vi "Main.vi"(11 "Module Admin":refnum<class "Delacor_lib_QMH_Module Admin.lvclass">) -> ()   [LabVIEW 2025, in "Automatic Teller Machine (ATM).lvlib"]
doc: "This template is based off of the Queued Message Handler design pattern and the Queued Message Handler project template that ships with LabVIEW.\n\nThe main difference is that the queue is private to this module and communication between modules is performed via Broadcast and Request events.\n\nRequest events are wrapped in public API methods and are handled in the Event Handling Loop (EHL) of this VI. Any module can register for Broadcast events sent by this module. The EHL generates messages based on user interface actions.\n\nThe Message Handling Loop (MHL) processes messages generated by the EHL, or by other messages. The messages are string values, so new messages can be added easily to the Message Cases case structure in the MHL. Each message cluster can also provide an optional value for Message Data, which is a variant that can be converted to whatever message-specific data is required.\n_____\nBased on DQMH Dev Tools: Project Template 7.1.0.1503."
uses:
  Automatic Teller Machine (ATM).lvlib
  <vilib>/Delacor/Delacor QMH/Libraries/Module Admin_class/Delacor_lib_QMH_Module Admin.lvclass
  Module Data--cluster.ctl
  <vilib>/Delacor/Delacor QMH/Libraries/Message Queue_class/Delacor_lib_QMH_Message Queue.lvclass/Delacor_lib_QMH_Message Queue.ctl
  Stop Argument--cluster.ctl
  <vilib>/Delacor/Delacor QMH/Libraries/Module Admin_class/Delacor_lib_QMH_Module Admin.lvclass/Delacor_lib_QMH_Module Admin.ctl
  Reset Timer Argument--cluster.ctl
  <vilib>/Utility/miscctls.llb/LVPointTypeDef.ctl
  <vilib>/Delacor/Delacor QMH/Libraries/Message Queue_class/Delacor_lib_QMH_Enqueue Message (Single).vi
  <vilib>/Delacor/Delacor QMH/Libraries/Module Admin_class/Delacor_lib_QMH_Get External Launch.vi
  <vilib>/Delacor/Delacor QMH/Libraries/Message Queue_class/Delacor_lib_QMH_Message Queue.lvclass
panel:
  in  "Enter":bool
  in  "User Input":string
  in  "Right Buttons":T1
  out "Right Menu":T2
  in  "Left Buttons":T1
  out "Left Menu":T2
  in  "Card Simulator":bool
  out "ATM Messages":string
  out "error out":errorcluster
  out "Status":string
  in  "Simulate MHL Error":bool
  in  "Simulate EHL Error":bool
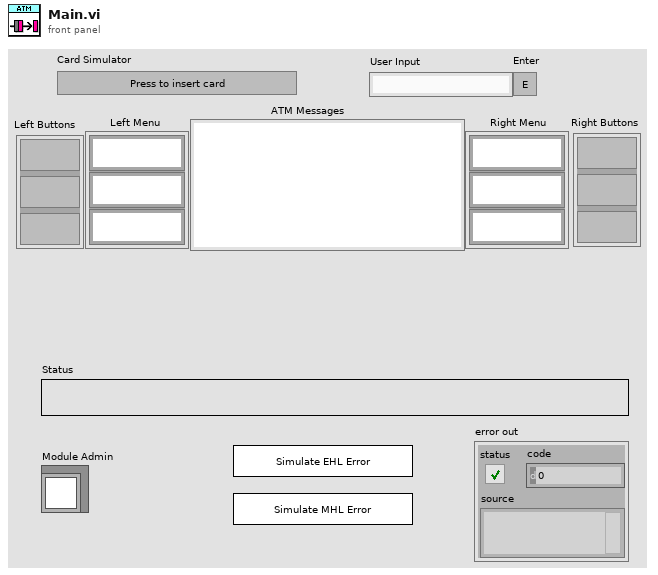
[diagram p1: front panel]
types:
  T1 = cluster{"Func Button":bool, "Func Button 2":bool, "Func Button 3":bool}
  T2 = cluster{"RFS String":string, "RFS String 2":string, "RFS String 3":string}
  T3 = typedef "Automatic Teller Machine (ATM).lvlib/Request Events--cluster.ctl" = cluster{"Stop Module":refnum<user-event>, "Show Panel":refnum<user-event>, "Hide Panel":refnum<user-event>, "Get Module Execution Status":refnum<user-event>, "Show Diagram":refnum<user-event>, "Private.Reset Timer":refnum<user-event>}
  T4 = typedef "Automatic Teller Machine (ATM).lvlib/Module Data--cluster.ctl" = cluster{"Status":string}
  T5 = enum32{"invalid lock state", "Not Locked", "Locked (No Password)", "Password-protected"}
  T6 = typedef "Automatic Teller Machine (ATM).lvlib/Stop Argument--cluster.ctl" = cluster{"Origin":string, "Exit via Stop Module Req?":bool, "Wait for Module to stop?":bool}
  T7 = typedef "Automatic Teller Machine (ATM).lvlib/Reset Timer Argument--cluster.ctl" = cluster{"Boolean":bool}
  T8 = typedef "LVPointTypeDef.ctl" = cluster{"Horizontal":i16, "Vertical":i16}
  T9 = enum32{"Invalid", "Standard", "Closed", "Hidden", "Minimized", "Maximized"}
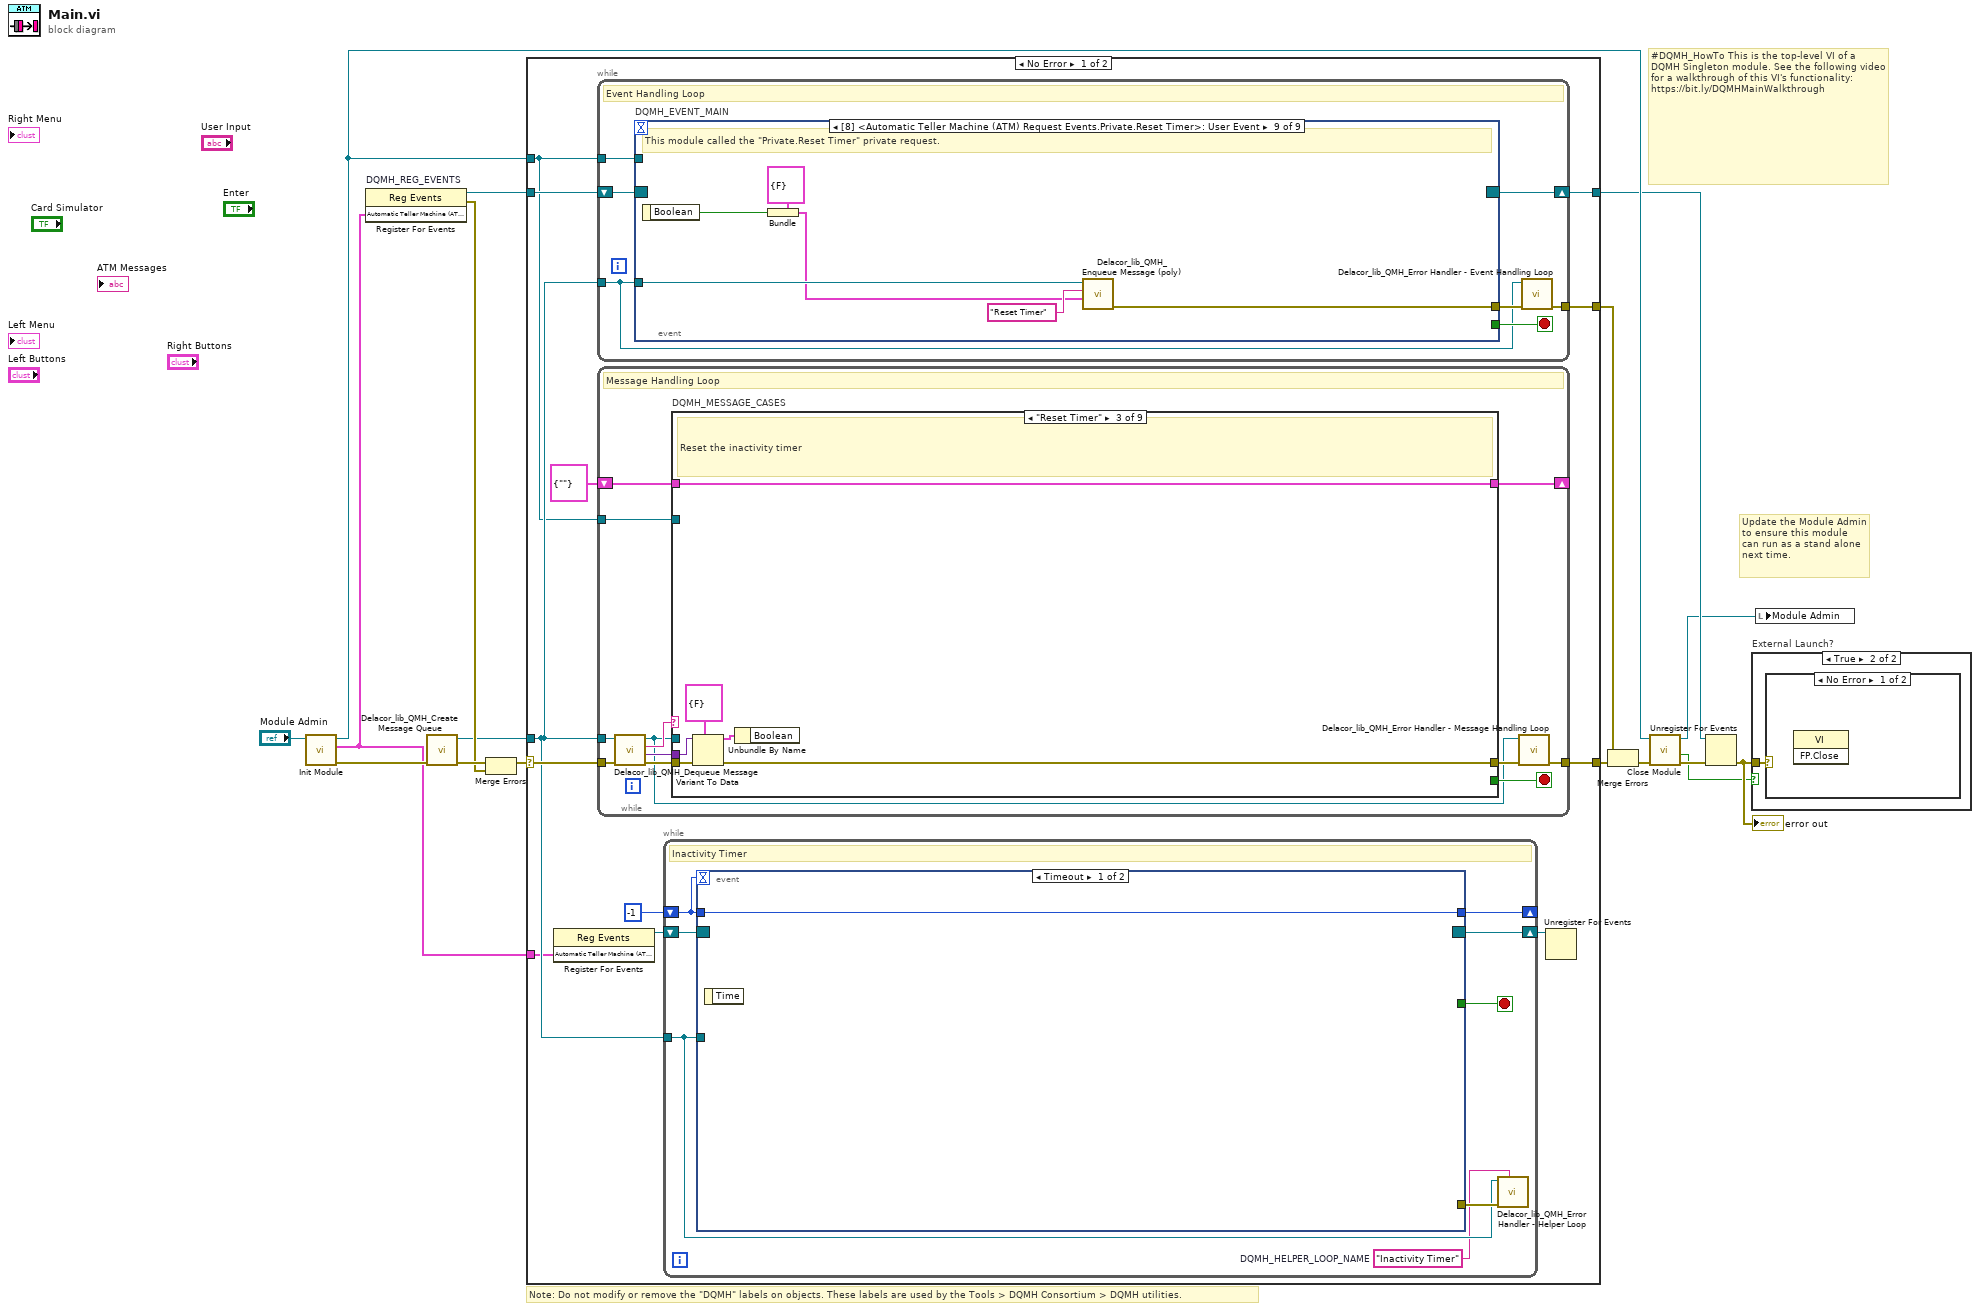
[diagram p0: block diagram]
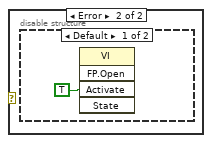
[diagram p3: hidden frame]
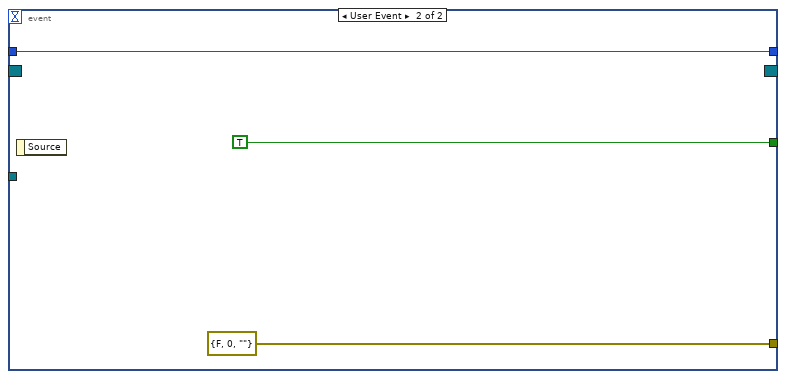
[diagram p5: hidden frame]
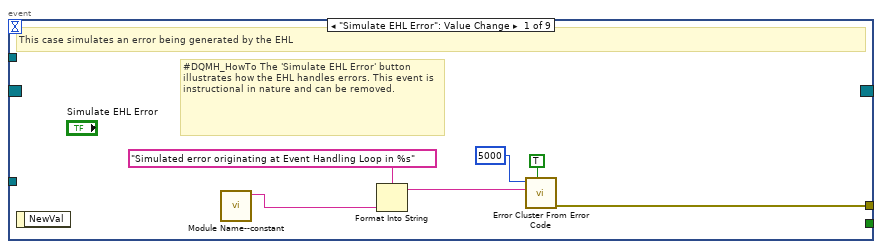
[diagram p6: hidden frame]
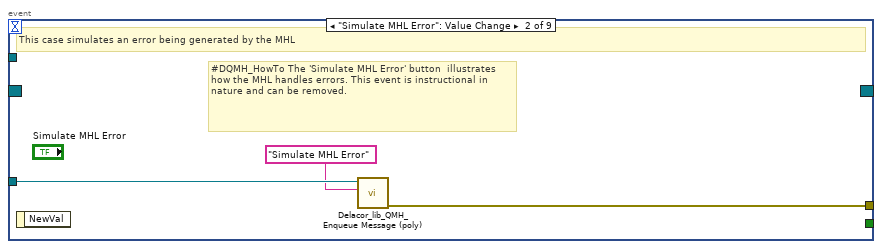
[diagram p7: hidden frame]
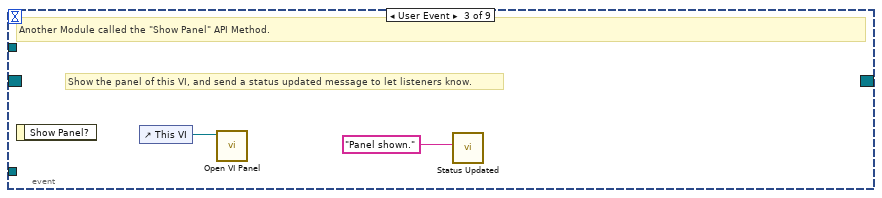
[diagram p8: hidden frame]
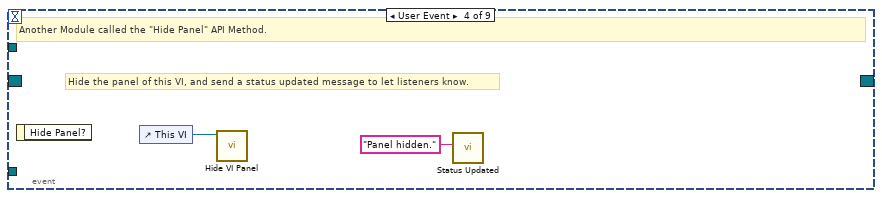
[diagram p9: hidden frame]
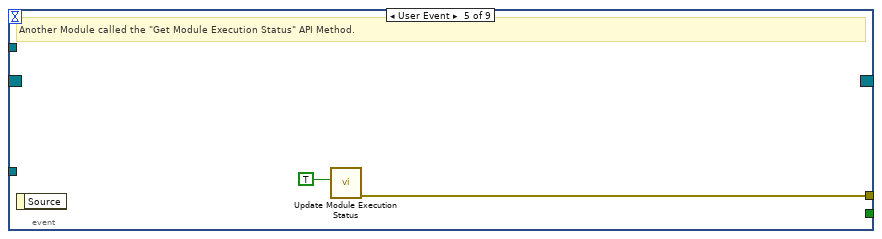
[diagram p10: hidden frame]
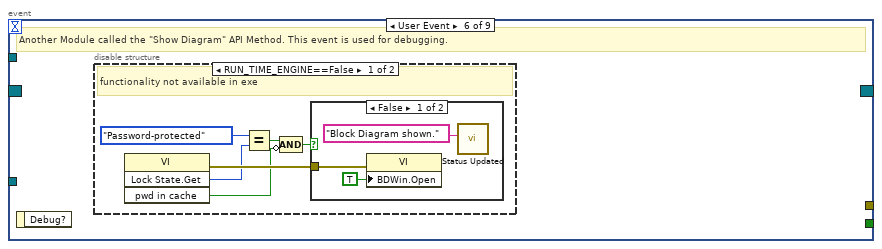
[diagram p11: hidden frame]
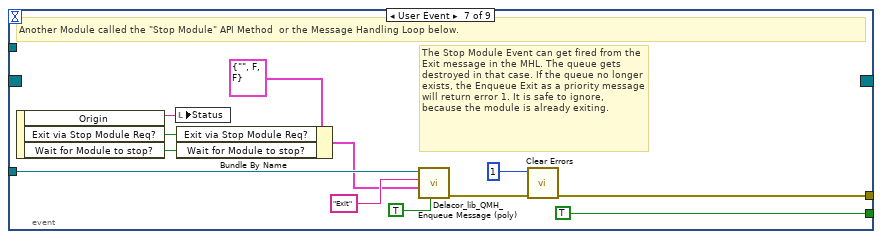
[diagram p14: hidden frame]
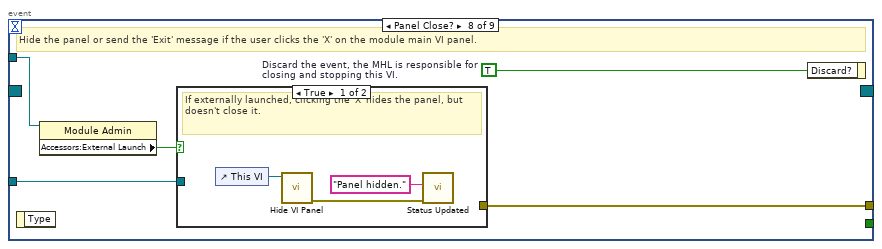
[diagram p15: hidden frame]
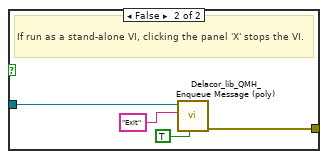
[diagram p16: hidden frame]
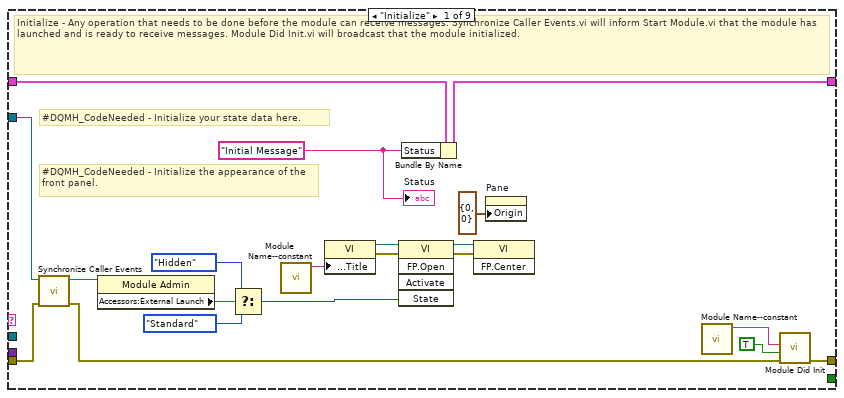
[diagram p17: hidden frame]
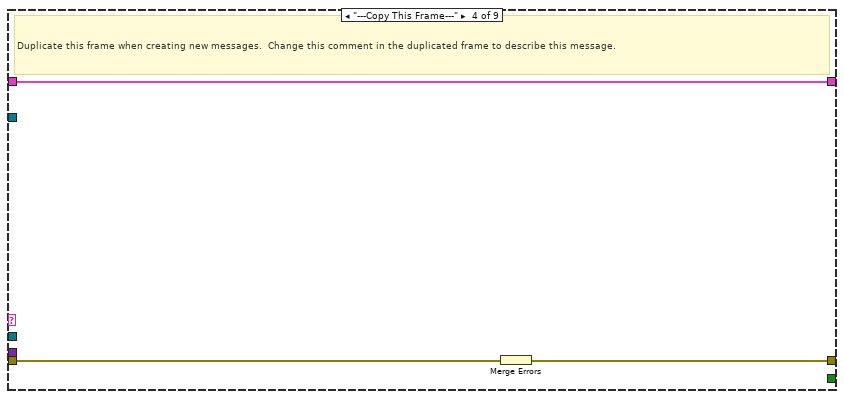
[diagram p19: hidden frame]
diagram:
  # "#DQMH_HowTo This is the top-level VI of a DQMH Singleton module. See the following video for a walkthrough of this VI's functionality: https://bit.ly/DQMHMainWalkthrough"
  # "Note: Do not modify or remove the \"DQMH\" labels on objects. These labels are used by the Tools > DQMH Consortium > DQMH utilities."
  # "Update the Module Admin to ensure this module can run as a stand alone next time."
  n1 = call "Init Module.vi"("Singleton Module Admin in"="Module Admin") -> ("error out"=w16:errorcluster, "Automatic Teller Machine (ATM) Request Events"=w1:T3, "Singleton Module Admin out"=w8:refnum<class "Delacor_lib_QMH_Module Admin.lvclass">)  [unwired: 8 in]
  n2 = register-events "DQMH_REG_EVENTS"(w1) -> (reference out=w6:refnum<event-registration>, error out=w9:errorcluster)  [unwired: 2 in]
  n3 = call <vilib>:"Delacor_lib_QMH_Create Message Queue.vi"("error in"=w16) -> ("error out"=w11:errorcluster, "Message Queue"=w5:refnum<class "Delacor_lib_QMH_Message Queue.lvclass">)  [unwired: 9 in]
  n4 = Merge Errors(w11, w9) -> (w10:errorcluster)
  n5 = case shown="No Error" w10 {
    selector: w10 -> [w27 w206]
    tunnel: [w29 w205] -> w17
    tunnel: [w26 w204] -> w7
    tunnel: w6 -> [w24 w204]
    tunnel: w5 -> [w23 w199]
    tunnel: [w28 _] -> w14
    tunnel: w8 -> [w22 w200]
    tunnel: w1 -> [w21 _]
    frame No Error {
      n6 = register-events ("DQMH_HELPER_REGFOREVENTS")(w21) -> (reference out=w19:refnum<event-registration>)  [unwired: 2 in, 1 out]
      n7 = while {
        tunnel: w23 -> [w42]
        shift-right: [w45] -> w26
        shift-left: w24 -> [w46]
        tunnel: [w47] -> w28
        tunnel: w22 -> [w43]
        stop <- w44 stop-if-true
        # "Event Handling Loop"
        n8 = event "DQMH_EVENT_MAIN" shown="[8] <Automatic Teller Machine (ATM) Request Events.Private.Reset Timer>: User Event" {
          selector: w46 -> [_ _ _ _ _ _ _ _ _]
          dyn-events: [_ _ _ _ _ _ _ _ _] -> w45
          timeout: _ -> [_ _ _ _ _ _ _ _ _]
          tunnel: [_ _ _ _ _ _ TRUE ("Discard?") _ _] -> w44
          tunnel: w42 -> [_ w56 _ _ _ _ w80 w87 w102]
          tunnel: [w54 w57 _ _ w63 _ w83 w89 w97] -> w48
          tunnel: w43 -> [_ _ _ _ _ _ _ w86 _]
          event "Simulate EHL Error": Value Change {
            # "#DQMH_HowTo The 'Simulate EHL Error' button  illustrates how the EHL handles errors. This event is instructional in nature and can be removed."
            # "This case simulates an error being generated by the EHL"
            n9 = event-data() -> ()  [unwired: 1 in, 1 out]
            n10 = call "Module Name--constant.vi"() -> ("Module Name"=w51:string)  [unwired: 11 in]
            n11 = Format Into String(format string="Simulated error originating at Event Handling Loop in %s", w51) -> (resulting string=w52:string)  [unwired: 2 in, 1 out]
            n12 = call <vilib>:"Error Cluster From Error Code.vi"("show call chain? (False)"=TRUE, "error message (\"\")"=w52, "error code (0)"=5000) -> ("error out"=w54:errorcluster)  [unwired: 6 in]
          }
          event "Simulate MHL Error": Value Change {
            # "#DQMH_HowTo The 'Simulate MHL Error' button  illustrates how the MHL handles errors. This event is instructional in nature and can be removed."
            # "This case simulates an error being generated by the MHL"
            n13 = event-data() -> ()  [unwired: 1 in, 1 out]
            n14 = call-poly <vilib>:"Delacor_lib_QMH_Enqueue Message (poly).vi"("Message"="Simulate MHL Error", "Message Queue in"=w56) -> ("error out"=w57:errorcluster)  [unwired: 8 in, 1 out]
          }
          event User Event {
            # "Show the panel of this VI, and send a status updated message to let listeners know."
            # "Another Module called the \"Show Panel\" API Method."
            n15 = event-data() -> ()  [unwired: 1 in, 1 out]
            n16 = control-ref of="This VI"() -> (w59:refnum<vi>)
            n17 = call "Open VI Panel.vi"("VI"=w59) -> ()  [unwired: 10 in, 1 out]
            n18 = call "Status Updated.vi"("Status"="Panel shown." ("format string")) -> ()  [unwired: 10 in, 1 out]
          }
          event User Event {
            # "Hide the panel of this VI, and send a status updated message to let listeners know."
            # "Another Module called the \"Hide Panel\" API Method."
            n19 = event-data() -> ()  [unwired: 1 in, 1 out]
            n20 = control-ref of="This VI"() -> (w61:refnum<vi>)
            n21 = call "Hide VI Panel.vi"("VI"=w61) -> ()  [unwired: 10 in, 1 out]
            n22 = call "Status Updated.vi"("Status"="Panel hidden." ("format string")) -> ()  [unwired: 10 in, 1 out]
          }
          event User Event {
            # "Another Module called the \"Get Module Execution Status\" API Method."
            n23 = event-data() -> ()  [unwired: 1 in, 1 out]
            n24 = call "Update Module Execution Status.vi"("Running?"=TRUE) -> ("error out"=w63:errorcluster)  [unwired: 10 in]
          }
          event User Event {
            # "Another Module called the \"Show Diagram\" API Method. This event is used for debugging."
            n25 = event-data() -> ()  [unwired: 1 in, 1 out]
            n26 = disable-structure shown="RUN_TIME_ENGINE==False" {
              frame condition #0 (active) {
                # "functionality not available in exe"
                n27 = invoke on="Invoke Node" class="VI" method="Lock State.Get"() -> (error out=w69:errorcluster, "Get Lock State"=w68:T5, "pwd in cache"=w65:bool)  [unwired: 4 in, 1 out]
                n28 = Equal?(x=T5."Password-protected", y=w68) -> (x = y?=w66:bool)
                n29 = Compound Arithmetic op=AND(w66, invert w65) -> (w64:bool)
                n30 = case shown="False" w64 {
                  tunnel: w69 -> [w72 _]
                  frame False {
                    n31 = property on="Property Node" class="VI"(error in=w72, "BDWin.Open"=TRUE ("Block Diagram Window:Open")) -> ()  [unwired: 1 in, 2 out]
                    n32 = call "Status Updated.vi"("Status"="Block Diagram shown." ("format string")) -> ()  [unwired: 10 in, 1 out]
                  }
                  frame True {
                    # "Password-protected VI, and the password is not in the cache. Do not show the diagram."
                  }
                }
              }
              frame condition #1 {
              }
            }
          }
          event User Event {
            # "The Stop Module Event can get fired from the Exit message in the MHL. The queue gets destroyed in that case. If the queue no longer exists, the Enqueue Exit as a priority message will return error 1. It is safe to ignore, because the module is already exiting."
            # "Another Module called the \"Stop Module\" API Method  or the Message Handling Loop below."
            n33 = event-data() -> ("Origin"=w79:string, "Exit via Stop Module Req?"=w75:bool, "Wait for Module to stop?"=w74:bool)  [unwired: 1 in]
            n34 = local write "Status"(w79) -> ()
            n35 = Bundle By Name(cluster=T6 {"Origin"="", "Exit via Stop Module Req?"=FALSE, "Wait for Module to stop?"=FALSE} ("Stop Argument"), "Exit via Stop Module Req?"=w75, "Wait for Module to stop?"=w74) -> (w73:T6)
            n36 = call-poly <vilib>:"Delacor_lib_QMH_Enqueue Message (poly).vi"("Priority Message? (F)"=TRUE, "Message Data"=w73, "Message"="Exit", "Message Queue in"=w80) -> ("error out"=w84:errorcluster)  [unwired: 6 in, 1 out]
            n37 = call <vilib>:"Clear Errors.vi"("error in (no error)"=w84, "specific error code to clear (0: all)"=1) -> ("error out"=w83:errorcluster)  [unwired: 4 in, 1 out]
          }
          event Panel Close? {
            w88 = TRUE  # Discard the event, the MHL is responsible for closing and stopping this VI.
            # "Hide the panel or send the 'Exit' message if the user clicks the 'X' on the module main VI panel."
            n38 = event-data() -> ()  [unwired: 1 in, 1 out]
            n39 = property on="Property Node" class="Module Admin"(reference=w86) -> ("Accessors:External Launch"=w85:bool)  [unwired: 1 in, 2 out]
            n40 = case shown="True" w85 {
              tunnel: w87 -> [_ w95]
              tunnel: [_ w96] -> w89
              frame True {
                # "If externally launched, clicking the 'X' hides the panel, but doesn't close it."
                n41 = control-ref of="This VI"() -> (w92:refnum<vi>)
                n42 = call "Hide VI Panel.vi"("VI"=w92) -> ("error out"=w90:errorcluster)  [unwired: 10 in]
                n43 = call "Status Updated.vi"("error in"=w90, "Status"="Panel hidden." ("format string")) -> ()  [unwired: 9 in, 1 out]
              }
              frame False {
                # "If run as a stand-alone VI, clicking the panel 'X' stops the VI."
                n44 = call-poly <vilib>:"Delacor_lib_QMH_Enqueue Message (poly).vi"("Priority Message? (F)"=TRUE, "Message"="Exit", "Message Queue in"=w95) -> ("error out"=w96:errorcluster)  [unwired: 7 in, 1 out]
              }
            }
            n45 = event-data ("Event Filter Node")("Discard?"=w88) -> ()  [unwired: 1 in, 1 out]
          }
          event User Event {
            # "This module called the \"Private.Reset Timer\" private request."
            n46 = event-data() -> ("Boolean"=w98:bool)  [unwired: 1 in]
            n47 = Bundle(cluster=T7 {"Boolean"=FALSE} ("Reset Timer Argument"), "Boolean"=w98) -> (w99:T7)
            n48 = call-poly <vilib>:"Delacor_lib_QMH_Enqueue Message (poly).vi"("Message Data"=w99, "Message"="Reset Timer", "Message Queue in"=w102) -> ("error out"=w97:errorcluster)  [unwired: 7 in, 1 out]
          }
        }
        n49 = call-dynamic "Delacor_lib_QMH_Error Handler - Event Handling Loop.vi"("error in"=w48, "Message Queue in"=w42) -> ("dup error in"=w47:errorcluster)  [unwired: 8 in, 1 out]
      }
      n50 = while {
        tunnel: w23 -> [w103]
        shift-right: [w111] -> _
        shift-left: T4 {"Status"=""} ("Data Cluster") -> [w112]
        tunnel: w27 -> [w114]
        tunnel: [w106] -> w29
        tunnel: w22 -> [w107]
        stop <- w110 stop-if-true
        # "Message Handling Loop"
        n51 = call-dynamic "Delacor_lib_QMH_Dequeue Message.vi"("error in"=w114, "Message Queue in"=w103) -> ("error out"=w113:errorcluster, "Message Data"=w108:variant, "Message"=w109:string, "Message Queue out"=w104:refnum<class "Delacor_lib_QMH_Message Queue.lvclass">)  [unwired: 6 in]
        n52 = case "DQMH_MESSAGE_CASES" shown="\"Reset Timer\"" w109 {
          selector: w109 -> [_ _ _ _ _ _ _ _ w194]
          tunnel: w104 -> [_ _ _ _ _ _ w160 w182 _]
          tunnel: w113 -> [w132 w136 w142 w145 w147 w156 w167 w188 w197]
          tunnel: [w130 w136 w140 w144 w147 w155 w163 w183 w198] -> w105
          tunnel: w112 -> [w121 w135 w141 w143 w146 w153 w162 w181 w195]
          tunnel: [w120 w135 w141 w143 w146 w153 w162 w181 w195] -> w111
          tunnel: [_ _ _ _ _ _ _ w180 _] -> w110
          tunnel: w108 -> [_ _ w139 _ _ _ w161 w179 _]
          tunnel: w107 -> [w122 _ _ _ _ _ w159 w174 _]
          frame "Initialize" {
            w116 = "Initial Message" ("Initial Message")
            # "#DQMH_CodeNeeded - Initialize the appearance of the front panel."
            # "#DQMH_CodeNeeded - Initialize your state data here."
            # "Initialize - Any operation that needs to be done before the module can receive messages. Synchronize Caller Events.vi will inform Start Module.vi that the module has launched and is ready to receive messages. Module Did Init.vi will broadcast that the module initialized."
            n53 = call "Synchronize Caller Events.vi"("error in"=w132, "Singleton Module Admin in"=w122) -> ("error out"=w131:errorcluster, "Singleton Module Admin out"=w117:refnum<class "Delacor_lib_QMH_Module Admin.lvclass">)  [unwired: 8 in]
            n54 = property on="Property Node" class="Module Admin"(reference=w117) -> ("Accessors:External Launch"=w126:bool)  [unwired: 1 in, 2 out]
            n55 = Select(t=T9."Hidden" ("State"), s=w126, f=T9."Standard" ("State")) -> (s? t:f=w123:T9)
            n56 = call "Module Name--constant.vi"() -> ("Module Name"=w129:string)  [unwired: 11 in]
            n57 = property on="Property Node" class="VI"("Front Panel.Title"=w129) -> (reference out=w128:refnum<vi>, error out=w134:errorcluster)  [unwired: 2 in]
            n58 = invoke on="Invoke Node" class="VI" method="FP.Open"(reference=w128, error in=w134, "State"=w123) -> (reference out=w127:refnum<vi>, error out=w133:errorcluster)  [unwired: 2 in, 3 out]
            n59 = Bundle By Name(cluster=w121, "Status"=w116) -> (w120:T4)
            n60 = invoke on="Invoke Node" class="VI" method="FP.Center"(reference=w127, error in=w133) -> ()  [unwired: 1 in, 3 out]
            n61 = property on="Pane" class="Pane"("Origin"=T8 {"Horizontal"=0, "Vertical"=0}) -> ()  [unwired: 2 in, 2 out]
            n62 = call "Module Name--constant.vi"() -> ("Module Name"=w118:string)  [unwired: 11 in]
            n63 = call "Module Did Init.vi"("error in"=w131, "Initialized?"=TRUE, "Origin"=w118) -> ("error out"=w130:errorcluster)  [unwired: 8 in]
            "Status" <- w116
          }
          frame "---Module Specific---" {
            # "Separator -- The following cases handle messages specific to this Module."
          }
          frame "Reset Timer" {
            # "Reset the inactivity timer"
            n64 = Variant To Data(error in=w142, type=T7 {"Boolean"=FALSE} ("Reset Timer Argument"), Variant=w139) -> (data=w137:T7, error out=w140:errorcluster)
            n65 = Unbundle By Name(w137) -> ()  [unwired: 1 out]
          }
          frame "---Copy This Frame---" {
            # "Duplicate this frame when creating new messages.  Change this comment in the duplicated frame to describe this message."
            n66 = Merge Errors(w145) -> (w144:errorcluster)
          }
          frame "---Exit and Error Handling---" {
            # "Separator - The following cases handle errors and exit messages."
          }
          frame "Simulate MHL Error" {
            # "#DQMH_HowTo The 'Simulate MHL Error' button  illustrates how the MHL handles errors. This event is instructional in nature and can be removed."
            # "Simulate an error occurring at the MHL"
            n67 = call "Module Name--constant.vi"() -> ("Module Name"=w149:string)  [unwired: 11 in]
            n68 = Format Into String(format string="Simulated error originating at Message Handling Loop in %s", w149) -> (resulting string=w150:string)  [unwired: 2 in, 1 out]
            n69 = call <vilib>:"Error Cluster From Error Code.vi"("show call chain? (False)"=TRUE, "error message (\"\")"=w150, "error code (0)"=5001) -> ("error out"=w154:errorcluster)  [unwired: 6 in]
            n70 = Merge Errors(w156, w154) -> (w155:errorcluster)
          }
          frame "Error" {
            # "#DQMH_CodeRecommended - If the module is running in standalone mode (External Launch = FALSE), this code will pop up an error dialog and call the 'Exit' message if an error occurs. Add more fine-grained error management here."
            # "Error - Check the error message data and respond accordingly. This message is sent by the \"Error Handler\" VIs at the end of each loop in this application."
            n71 = property on="Property Node" class="Module Admin"(reference=w159) -> ("Accessors:External Launch"=w158:bool)  [unwired: 1 in, 2 out]
            n72 = Variant To Data(error in=w167, type=errorcluster {"status"=FALSE, "code"=0, "source"=""} ("error constant"), Variant=w161) -> (data=w157:errorcluster, error out=w165:errorcluster)
            n73 = local write "error out"(w157) -> ()
            n74 = call "Error Reported.vi"("Error"=w157) -> ()  [unwired: 10 in, 1 out]
            n75 = case shown="False" w158 {
              tunnel: [w172 _] -> w164
              tunnel: w160 -> [w170 _]
              tunnel: w157 -> [w171 _]
              frame False {
                n76 = disable-structure shown="Default" {
                  disable-tunnel: w171 -> [w173 _]
                  frame condition #0 (active) {
                    # "If the module is running standalone, then pop up an error dialog and call the \"Exit\" message."
                    n77 = call <vilib>:"Simple Error Handler.vi"("error in (no error)"=w173) -> ()  [unwired: 4 in, 5 out]
                  }
                  frame condition #1 {
                    # "To prevent the Simple Error Handler VI from being loaded (e.g. when deploying to a Real-Time target), add the Conditional Disable Symbol \"DQMH_Disable_SEH\" to your project and set it to TRUE."
                  }
                }
                n78 = call-poly <vilib>:"Delacor_lib_QMH_Enqueue Message (poly).vi"("Priority Message? (F)"=TRUE, "Message"="Exit", "Message Queue in"=w170) -> ("error out"=w172:errorcluster)  [unwired: 7 in, 1 out]
              }
              frame True {
                # "If the module was launched externally, calling the Error Reported broadcast VI is the only action performed by the \"Error\" message. The module's caller can then process the error appropriately."
              }
            }
            n79 = Merge Errors(w165, w164) -> (w163:errorcluster)
          }
          frame "Exit" {
            w178 = 91  # 91: not all Exit messages will have an argument
            w180 = TRUE  # Stop the VI
            # "Release the message queue reference"
            # "#DQMH_CodeNeeded - Add any required cleanup code here."
            # "Exit - Exit the application."
            n80 = Variant To Data(error in=w188, type=T6 {"Origin"="", "Exit via Stop Module Req?"=FALSE, "Wait for Module to stop?"=FALSE} ("Stop Argument"), Variant=w179) -> (data=w176:T6, error out=w185:errorcluster)
            n81 = call <vilib>:"Clear Errors.vi"("error in (no error)"=w185, "specific error code to clear (0: all)"=w178) -> ("error out"=w187:errorcluster)  [unwired: 4 in, 1 out]
            n82 = control-ref of="This VI"() -> (w175:refnum<vi>)
            n83 = call-dynamic "Delacor_lib_QMH_Release Message Queue.vi"("error in"=w187, "Message Queue"=w182) -> ("error out"=w186:errorcluster)  [unwired: 9 in]
            n84 = call "Handle Exit.vi"("Stop Argument"=w176, "Admin in"=w174, "VI reference"=w175) -> ("error out"=w184:errorcluster)  [unwired: 7 in, 1 out]
            n85 = Merge Errors(w186, w184) -> (w183:errorcluster)
            n86 = call "Error Reported.vi"("Error"=w183) -> ()  [unwired: 10 in, 1 out]
          }
          frame Default {
            # "'Default' case only runs if there is a message that isn't defined in any of the other cases.  Output a programming error."
            n87 = call "Module Name--constant.vi"() -> ("Module Name"=w193:string)  [unwired: 11 in]
            n88 = Format Into String(format string="The invalid message string \"%s\" was received in the Message Handling Loop for module \"%s\".", w194, w193) -> (resulting string=w189:string)  [unwired: 2 in, 1 out]
            n89 = call <vilib>:"Error Cluster From Error Code.vi"("show call chain? (False)"=TRUE, "error message (\"\")"=w189, "error code (0)"=1) -> ("error out"=w196:errorcluster)  [unwired: 6 in]
            n90 = Merge Errors(w197, w196) -> (w198:errorcluster)
          }
        }
        n91 = call-dynamic "Delacor_lib_QMH_Error Handler - Message Handling Loop.vi"("error in"=w105, "Message Queue in"=w104) -> ("dup error in"=w106:errorcluster)  [unwired: 8 in, 1 out]
      }
      n92 = while "DQMH_HELPER_LOOP" {
        shift-right: [w37] -> _
        shift-left: -1 -> [w36]
        shift-right: [w34] -> w20
        shift-left: w19 -> [w35]
        tunnel: w23 -> [w31]
        stop <- w33 stop-if-true
        w30 = "Inactivity Timer"  # DQMH_HELPER_LOOP_NAME
        # "Inactivity Timer"
        n93 = event "DQMH_HELPER_EVENT_STRUCTURE" shown="[0] Timeout" {
          selector: w35 -> [_ _]
          dyn-events: [_ _] -> w34
          timeout: w36 -> [_ _]
          tunnel: w36 -> [w38 w41]
          tunnel: [w38 w41] -> w37
          tunnel: [_ TRUE] -> w33
          tunnel: [_ errorcluster {"status"=FALSE, "code"=0, "source"=""} ("error constant")] -> w32
          tunnel: w31 -> [_ _]
          event Timeout {
            n94 = event-data() -> ()  [unwired: 1 in, 1 out]
          }
          event User Event {
            n95 = event-data() -> ()  [unwired: 1 in, 1 out]
          }
        }
        n96 = call-dynamic "Delacor_lib_QMH_Error Handler - Helper Loop.vi"("Error Debug"=w30, "error in"=w32, "Message Queue in"=w31) -> ()  [unwired: 7 in, 2 out]
      }
      n97 = Unregister For Events(event registration refnum=w20) -> ()  [unwired: 1 in, 1 out]
    }
    frame Error {
      # "Synchronize Caller Events.vi will inform Start Module.vi that the module has launched and will let the code calling Start Module.vi register for broadcasts and would permit the caller receive the broadcast that an error occurred at launch time."
      n98 = call-dynamic "Delacor_lib_QMH_Release Message Queue.vi"("error in"=w206, "Message Queue"=w199) -> ("error out"=w205:errorcluster)  [unwired: 9 in]
      n99 = call "Synchronize Caller Events.vi"("Singleton Module Admin in"=w200) -> ("error out"=w207:errorcluster)  [unwired: 9 in, 1 out]
      n100 = call "Module Name--constant.vi"() -> ("Module Name"=w203:string)  [unwired: 11 in]
      n101 = Format Into String(format string="An error occurred during initialization. %s is no longer running.", w203) -> (resulting string=w201:string)  [unwired: 2 in, 1 out]
      n102 = Merge Errors(w205, w207) -> (w208:errorcluster)
      n103 = call "Error Reported.vi"("Additional Information"=w201, "Error"=w208) -> ()  [unwired: 9 in, 1 out]
    }
  }
  n104 = Merge Errors(w14, w17) -> (w13:errorcluster)
  n105 = call "Close Module.vi"("error in"=w13, "Module Admin in"=w8) -> ("error out"=w15:errorcluster, "External Launch"=w2:bool, "Module Admin out"=w3:refnum<class "Delacor_lib_QMH_Module Admin.lvclass">)  [unwired: 7 in]
  n106 = Unregister For Events(event registration refnum=w7, error in=w15) -> (error out=w12:errorcluster)
  "error out" <- w12
  n107 = case "External Launch?" shown="True" w2 {
    tunnel: w12 -> [_ w209]
    frame False {
    }
    frame True {
      n108 = case shown="No Error" w209 {
        frame No Error {
          n109 = invoke on="Invoke Node" class="VI" method="FP.Close"() -> ()  [unwired: 3 in, 3 out]
        }
        frame Error {
          n110 = disable-structure shown="Default" {
            frame condition #0 (active) {
              n111 = invoke class="VI" method="FP.Open"("Activate"=TRUE ("Activate?")) -> ()  [unwired: 4 in, 5 out]
            }
            frame condition #1 {
              # "Don't show panel on error if running inside a built EXE."
            }
          }
        }
      }
    }
  }
  n112 = local write "Module Admin"(w3) -> ()
